vi "Direction Position Offsets.vi"() -> (3 "Direction Position Offsets":T1[](array[typedef])=[{"Row"=1, "Col"=-1}, {"Row"=1, "Col"=0}, {"Row"=1, "Col"=1}, {"Row"=0, "Col"=1}, {"Row"=-1, "Col"=1}, {"Row"=-1, "Col"=0}, {"Row"=-1, "Col"=-1}, {"Row"=0, "Col"=-1}])   [LabVIEW 2020, in "SquareBattle.lvlib"]
uses:
  SquareBattle.lvlib
  Position.ctl
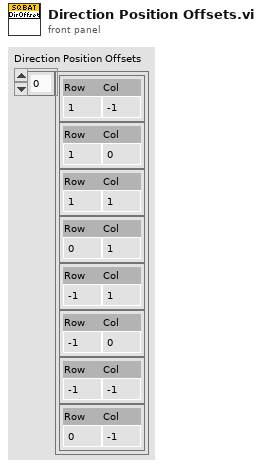
[diagram p1: front panel]
types:
  T1 = typedef "SquareBattle.lvlib/Position.ctl" = cluster{"Row":i32, "Col":i32}
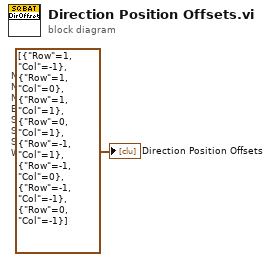
[diagram p0: block diagram]
diagram:
  # "NW\nN\nNE\nE\nSE\nS\nSW\nW"
  "Direction Position Offsets" <- T1[] [{"Row"=1, "Col"=-1}, {"Row"=1, "Col"=0}, {"Row"=1, "Col"=1}, {"Row"=0, "Col"=1}, {"Row"=-1, "Col"=1}, {"Row"=-1, "Col"=0}, {"Row"=-1, "Col"=-1}, {"Row"=0, "Col"=-1}] ("Array")
